vi "Update FSM State.vi"(8 "error in (no error)":errorcluster, 11 "FSM Data in":cluster{"FSM State":T1}) -> (0 "error out":errorcluster, 2 "FSM State":T1, 3 "FSM Data out":cluster{"FSM State":T1})   [LabVIEW 2016]
uses:
  FSM States.ctl
  Application Globals.vi
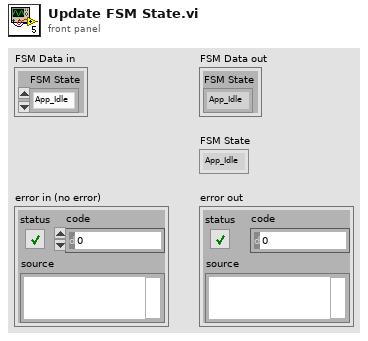
[diagram p1: front panel]
types:
  T1 = typedef "FSM States.ctl" = enum16{"App_Idle", "App_Connect", "App_Close", "APP_Init", "App_Logging", "App_SetRecordStateOn", "App_SetRecordStateOff"}
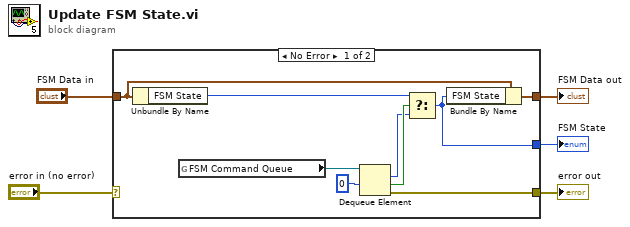
[diagram p0: block diagram]
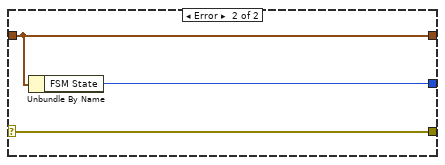
[diagram p2: hidden frame]
diagram:
  n1 = case shown="No Error" "error in (no error)" {
    selector: "error in (no error)" -> [_ w17]
    tunnel: "FSM Data in" -> [w9 w15]
    tunnel: [w8 w16] -> w2
    tunnel: [w7 w15] -> w3
    tunnel: [w6 w17] -> w4
    frame No Error {
      n2 = Unbundle By Name(w9) -> ("FSM State"=w10:T1)
      n3 = global read "Application Globals.vi" "FSM Command Queue"() -> (w14:refnum<queue>)
      n4 = Dequeue Element(queue=w14, timeout in ms (-1)=0) -> (element=w11:T1, timed out?=w12:bool, error out=w6:errorcluster)  [unwired: 1 in, 1 out]
      n5 = Select(t=w10, s=w12, f=w11) -> (s? t:f=w8:T1)
      n6 = Bundle By Name(cluster=w9, "FSM State"=w8) -> (w7:cluster{"FSM State":T1})
    }
    frame Error {
      n7 = Unbundle By Name(w15) -> ("FSM State"=w16:T1)
    }
  }
  "error out" <- w4
  "FSM Data out" <- w3
  "FSM State" <- w2
